vi "From String Array.vi"(8 "error in (no error)":errorcluster, 9 "String Array":string[](array[string]), 11 "Update Tag Config in":refnum<class "Update Tag Config.lvclass">) -> (0 "error out":errorcluster, 3 "Update Tag Config out":refnum<class "Update Tag Config.lvclass">)   [LabVIEW 2015, in "Update Tag Config.lvclass"]
uses:
  Update Tag Config.lvclass
  <vilib>/NI/Tag Bus Module Framework/channel/channel classification.ctl
  <vilib>/NI/Tag Bus/tag/Data Type.ctl
  <vilib>/NI/Tag Bus Module Framework/channel/TBM channel.lvclass
  <vilib>/NI/Tag Bus/tag/tag descriptor.lvclass
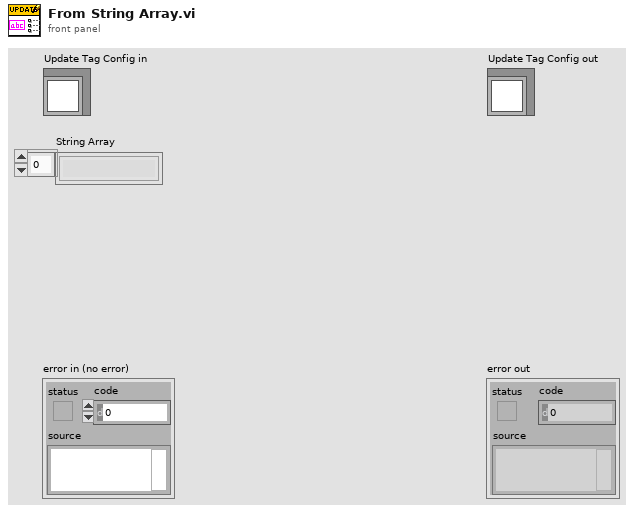
[diagram p1: front panel]
types:
  T1 = typedef "TBM channel.lvclass/channel classification.ctl" = enum16{"input data", "output data", "processing parameter", "processing result"}
  T2 = typedef "tag bus.lvlib/tag descriptor.lvclass/Data Type.ctl" = enum16{"Double", "Single", "I64", "I32", "I16", "I8", "U64", "U32", "U16", "U8", "Boolean", "String", "Array of Double", "Array of Single", "Array of I64", "Array of I32", "Array of I16", "Array of I8", "Array of U64", "Array of U32", "Array of U16", "Array of U8", "Array of Boolean", "Array of String"}
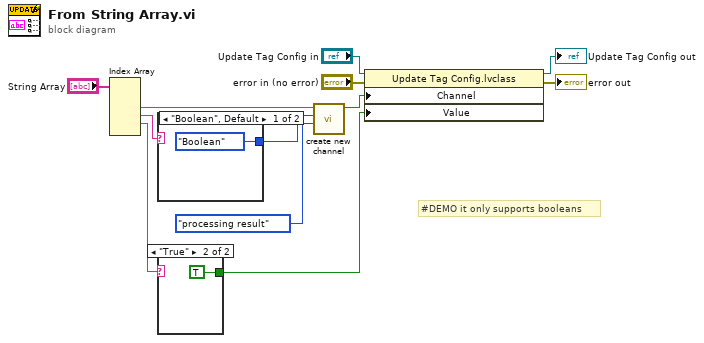
[diagram p0: block diagram]
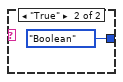
[diagram p3: hidden frame]
diagram:
  # "#DEMO it only supports booleans"
  n1 = Index Array(array="String Array") -> (element #2=w7:string, element #3=w6:string, element #4=w4:string)  [unwired: 5 in, 2 out]
  n2 = case shown="\"Boolean\", Default" w6 {
    tunnel: [Data_Type."Boolean" ("data type") Data_Type."Boolean" ("data type")] -> w5
    frame "Boolean", Default {
    }
    frame "True" {
    }
  }
  n3 = case shown="\"True\"" w4 {
    tunnel: [_ TRUE] -> w3
    frame "False", Default {
    }
    frame "True" {
    }
  }
  n4 = call <vilib>:"create new channel.vi"("channel classification"=channel_classification."processing result", "data type"=w5, "channel name"=w7) -> ("channel"=w2:refnum<class "TBM channel.lvclass">)  [unwired: 8 in]
  n5 = property class="Update Tag Config.lvclass"(reference="Update Tag Config in", error in="error in (no error)", "Channel"=w2, "Value"=w3) -> (reference out=→"Update Tag Config out":refnum<class "Update Tag Config.lvclass">, error out=→"error out":errorcluster)
